vi "SGUI Register Controls Groups.vi"(0 "control groups":T1(array[cluster]), 2 "error in":errorcluster, 6 "groups names":string, 8 "register mode (overwrite)":T2=enum."Overwrite", 10 "controls ID (empty)":string) -> (12 "assigned ID":string, 16 "error out":errorcluster)   [LabVIEW 2020, in "varilib.lvlib"]
doc: "This VI registers groups of controls for group control functions of SGUI lib. List of references is assigned together with name strings (multiline string, one line per group). Multiple groups are registered by single call. The primary use is for these functions is easy enabling/disabling of whole groups of controls by single command without listing them every time.\nI.e. for instance one group is stop button called 'busy', another group are buttons used for setup and start of some measurements called 'ready'. Later anywhere in the application the enable states of the controls can be changed by calling group function with 'busy' or 'ready' parameter. Number of groups is not limited. \n\nWhen sub-panel is displayed this VI can be called again to register new control groups. It can either overwrite originals or add new ones to stack. When the sub-panel is closed, thi VI may be called with 'release' parameter to remove last registered groups. Eventually 'Release ID' can be called to remove group by name ID.\n\nWhen called for the first time in the main VI is must be called with default 'overwrite' parameter in order to get rid of residue of data in the global variable of the SGUI lib!\n\nThis VI ignores input error and will not generate error."
uses:
  varilib.lvlib
  SGUI Global Var.vi
  <vilib>/ErrorRing/Error Ring.xnode
  <vilib>/Utility/error.llb/Error Cluster From Error Code.vi
  SGUI Assign References Mode.ctl
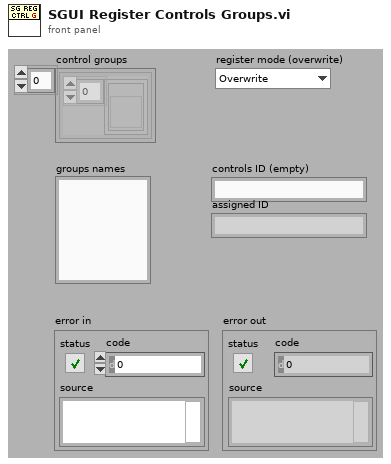
[diagram p1: front panel]
types:
  T1 = cluster{"control references (empty)":refnum<vi>[]}[]
  T2 = typedef "varilib.lvlib/SGUI Assign References Mode.ctl" = enum16{"Add to stack", "Overwrite", "Release last", "Release ID"}
  T3 = cluster{string[], cluster{"control references (empty)":refnum<vi>[]}[], "controls ID (empty)":string}
  T4 = cluster{"group names":string[], "controls per goups":cluster{"control references (empty)":refnum<vi>[]}[], "ID":string}[]
  T5 = cluster{string[], cluster{"control references (empty)":refnum<vi>[]}[], "controls ID (empty)":string}[]
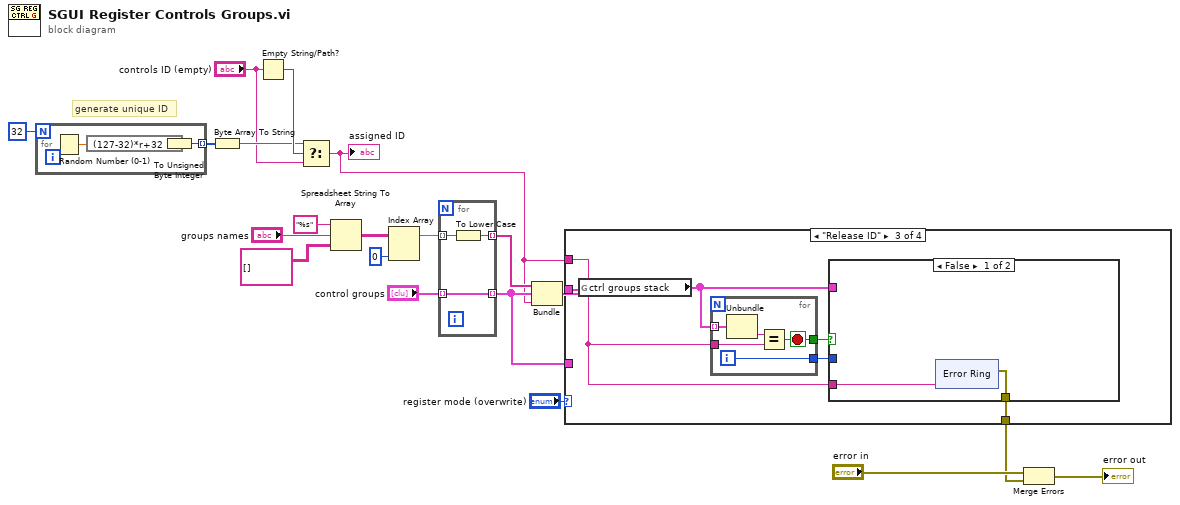
[diagram p0: block diagram]
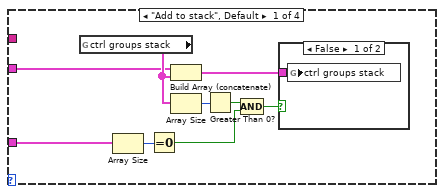
[diagram p2: hidden frame]
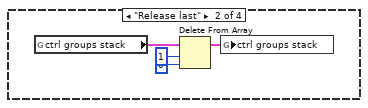
[diagram p4: hidden frame]
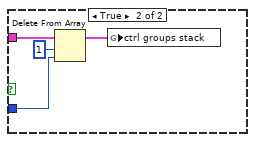
[diagram p5: hidden frame]
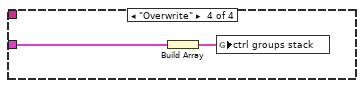
[diagram p6: hidden frame]
diagram:
  # "generate unique ID"
  n1 = for {
    N: 32 -> [_]
    tunnel: [w21] -> w9 mode=indexing
    n2 = Random Number (0-1)() -> (number: 0 to 1=w23:dbl)
    n3 = expression code="(127-32)*r+32"(w23) -> (w22:dbl)
    n4 = To Unsigned Byte Integer(number=w22) -> (unsigned 8bit integer=w21:u8)
  }
  n5 = Byte Array To String(unsigned byte array=w9) -> (string=w6:string)
  n6 = Empty String/Path?(string/path="controls ID (empty)") -> (empty?=w7:bool)
  n7 = Select(t=w6, s=w7, f="controls ID (empty)") -> (s? t:f=w4:string)
  "assigned ID" <- w4
  n8 = Spreadsheet String To Array(format string="%s", spreadsheet string="groups names", array type (2D Dbl)=string[][] []) -> (array=w15:string[][])  [unwired: 1 in]
  n9 = Index Array(array=w15, index (col)=0 ("disabled index (col)")) -> (element=w11:string[])  [unwired: 1 in]
  n10 = for {
    tunnel: "control groups" -> [w25] mode=indexing
    tunnel: w11 -> [w26] mode=indexing
    tunnel: [w24] -> w14 mode=indexing
    tunnel: [w25] -> w12 mode=indexing
    n11 = To Lower Case(string=w26) -> (all lower case string=w24:string)
  }
  n12 = Bundle(w14, w12, "controls ID (empty)"=w4) -> (w13:T3)  [unwired: 1 in]
  n13 = case shown="\"Release ID\"" "register mode (overwrite)" {
    tunnel: w13 -> [w28 _ _ w65]
    tunnel: w12 -> [w27 _ _ _]
    tunnel: w4 -> [_ _ w42 _]
    tunnel: [_ _ w41 _] -> w2
    frame "Add to stack", Default {
      n14 = global read "SGUI Global Var.vi" "ctrl groups stack"() -> (w31:T4)
      n15 = Array Size(array=w27) -> (size(s)=w29:i32)
      n16 = Equal To 0?(x=w29) -> (x = 0?=w33:bool)
      n17 = Build Array (concatenate)(w28, w31) -> (w30:T4)
      n18 = Array Size(array=w31) -> (size(s)=w35:i32)
      n19 = Greater Than 0?(x=w35) -> (x > 0?=w34:bool)
      n20 = Compound Arithmetic op=AND(w34, w33) -> (w32:bool)
      n21 = case shown="False" w32 {
        tunnel: w30 -> [w36 _]
        frame False {
          n22 = global write "SGUI Global Var.vi" "ctrl groups stack"(w36) -> ()
        }
        frame True {
        }
      }
    }
    frame "Release last" {
      n23 = global read "SGUI Global Var.vi" "ctrl groups stack"() -> (w40:T4)
      n24 = Delete From Array(array=w40, length=1, index=0) -> (array with subset deleted=w37:T4)  [unwired: 1 out]
      n25 = global write "SGUI Global Var.vi" "ctrl groups stack"(w37) -> ()
    }
    frame "Release ID" {
      n26 = global read "SGUI Global Var.vi" "ctrl groups stack"() -> (w43:T4)
      n27 = for {
        tunnel: w43 -> [w63] mode=indexing
        tunnel: w42 -> [w61]
        tunnel: [w60] -> w44
        tunnel: [w59] -> w45
        i -> [w60]
        stop <- w59 stop-if-true
        n28 = Unbundle(w63) -> ("ID"=w62:string)  [unwired: 2 out]
        n29 = Equal?(x=w62, y=w61) -> (x = y?=w59:bool)
      }
      n30 = case shown="False" w45 {
        tunnel: w44 -> [_ w56]
        tunnel: w43 -> [_ w58]
        tunnel: w42 -> [w47 _]
        tunnel: [w46 _] -> w41
        frame False {
          n31 = xnode "Error Ring"("parameter 0"=w47) -> ("error out"=w46:errorcluster)
        }
        frame True {
          n32 = Delete From Array(array=w58, length=1, index=w56) -> (array with subset deleted=w55:T4)  [unwired: 1 out]
          n33 = global write "SGUI Global Var.vi" "ctrl groups stack"(w55) -> ()
        }
      }
    }
    frame "Overwrite" {
      n34 = Build Array(w65) -> (w64:T5)
      n35 = global write "SGUI Global Var.vi" "ctrl groups stack"(w64) -> ()
    }
  }
  n36 = Merge Errors("error in", w2) -> (→"error out":errorcluster)
